vi "Scope_4c_Test2.vi"(8 "Channel 4":dbl, 9 "Channel 3":dbl, 10 "Channel 2":dbl, 11 "Channel 1":dbl) -> (3 "Display":waveform(dbl)[](graph) caption="伺服代码效率")   [LabVIEW 2015]
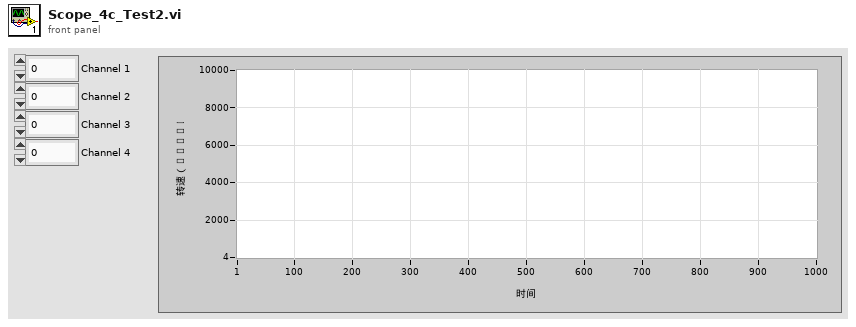
[diagram p1: front panel]
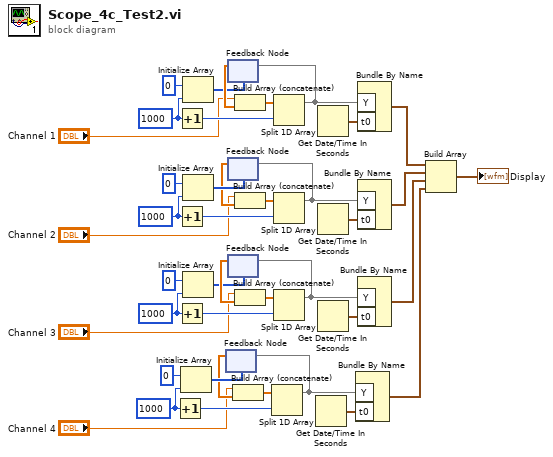
[diagram p0: block diagram]
diagram:
  w6 = 1000
  w19 = 1000
  w27 = 1000
  w36 = 1000
  n1 = Increment(x=w6) -> (x+1=w5:i32)
  n2 = Increment(x=w36) -> (x+1=w37:i32)
  n3 = Increment(x=w27) -> (x+1=w26:i32)
  n4 = Increment(x=w19) -> (x+1=w20:i32)
  n5 = Initialize Array(0, w6) -> (w9:i32[])
  n6 = Initialize Array(0, w36) -> (w33:i32[])
  n7 = Initialize Array(0, w27) -> (w30:i32[])
  n8 = Initialize Array(0, w19) -> (w16:i32[])
  n9 = feedback #1(w9) -> (w4:dbl[])
  n10 = feedback #2(w33) -> (w38:dbl[])
  n11 = feedback #3(w30) -> (w25:dbl[])
  n12 = feedback #4(w16) -> (w21:dbl[])
  n13 = Build Array (concatenate)("Channel 4", w4) -> (w7:dbl[])
  n14 = Build Array (concatenate)("Channel 1", w38) -> (w35:dbl[])
  n15 = Build Array (concatenate)("Channel 2", w25) -> (w28:dbl[])
  n16 = Build Array (concatenate)("Channel 3", w21) -> (w18:dbl[])
  n17 = Split 1D Array(array=w7, index=w5) -> (first subarray=w3:dbl[])  [unwired: 1 out]
  n18 = feedback-in #1(w3) -> ()
  n19 = Split 1D Array(array=w35, index=w37) -> (first subarray=w40:dbl[])  [unwired: 1 out]
  n20 = feedback-in #2(w40) -> ()
  n21 = Split 1D Array(array=w28, index=w26) -> (first subarray=w24:dbl[])  [unwired: 1 out]
  n22 = feedback-in #3(w24) -> ()
  n23 = Split 1D Array(array=w18, index=w20) -> (first subarray=w22:dbl[])  [unwired: 1 out]
  n24 = feedback-in #4(w22) -> ()
  n25 = Get Date/Time In Seconds() -> (seconds since 1Jan1904=w10:timestamp)
  n26 = Get Date/Time In Seconds() -> (seconds since 1Jan1904=w32:timestamp)
  n27 = Get Date/Time In Seconds() -> (seconds since 1Jan1904=w31:timestamp)
  n28 = Get Date/Time In Seconds() -> (seconds since 1Jan1904=w15:timestamp)
  n29 = Bundle By Name("Y"=w3, "t0"=w10) -> (w2:waveform(dbl))  [unwired: 1 in]
  n30 = Bundle By Name("Y"=w40, "t0"=w32) -> (w41:waveform(dbl))  [unwired: 1 in]
  n31 = Bundle By Name("Y"=w24, "t0"=w31) -> (w23:waveform(dbl))  [unwired: 1 in]
  n32 = Bundle By Name("Y"=w22, "t0"=w15) -> (w14:waveform(dbl))  [unwired: 1 in]
  n33 = Build Array(w41, w23, w14, w2) -> (→"Display":waveform(dbl)[])
